vi "test2-ProcessAsyncMessageWithReplyInCSMLoop(SendAndReceive).vi"(8 "error in (no error)":errorcluster, 11 "TestCase in":refnum<class "testcase-CSMAddonLoopSupport.lvclass">) -> (0 "error out":errorcluster, 3 "TestCase out":refnum<class "testcase-CSMAddonLoopSupport.lvclass">)   [LabVIEW 2017, in "testcase-CSMAddonLoopSupport.lvclass"]
uses:
  testcase-CSMAddonLoopSupport.lvclass
  4585ddd5-ba69-4fd4-94fe-207595864cbd.vi
  a7620e19-6451-46a1-85ca-ade5edb58587.vi
  55fec5d7-cd22-46f7-b641-2c7c49619fc8.vi
  9cfd6824-310a-46c9-9b98-3854de5c7aa2.vi
  <vilib>/addons/_JKI Toolkits/VI Tester/TestCase.llb/TestCase.lvclass
  src/user.lib/_NEVSTOP/Communicable State Machine(CSM)/Communicable State Machine.lvlib
  CSM/CSM-Testcase.lvlib
  C:/Program Files (x86)/National Instruments/LabVIEW 2017/vi.lib/addons/_JKI Toolkits/VI Tester/TestCase.llb/TestCase.lvclass
panel:
  out "LoopCount":i32
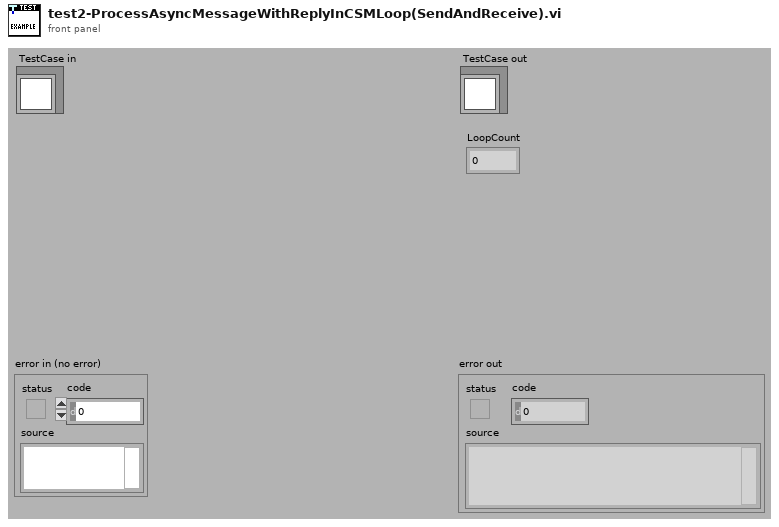
[diagram p1: front panel]
types:
  T1 = cluster{"Arguments":string, "Response":string, "error":errorcluster}
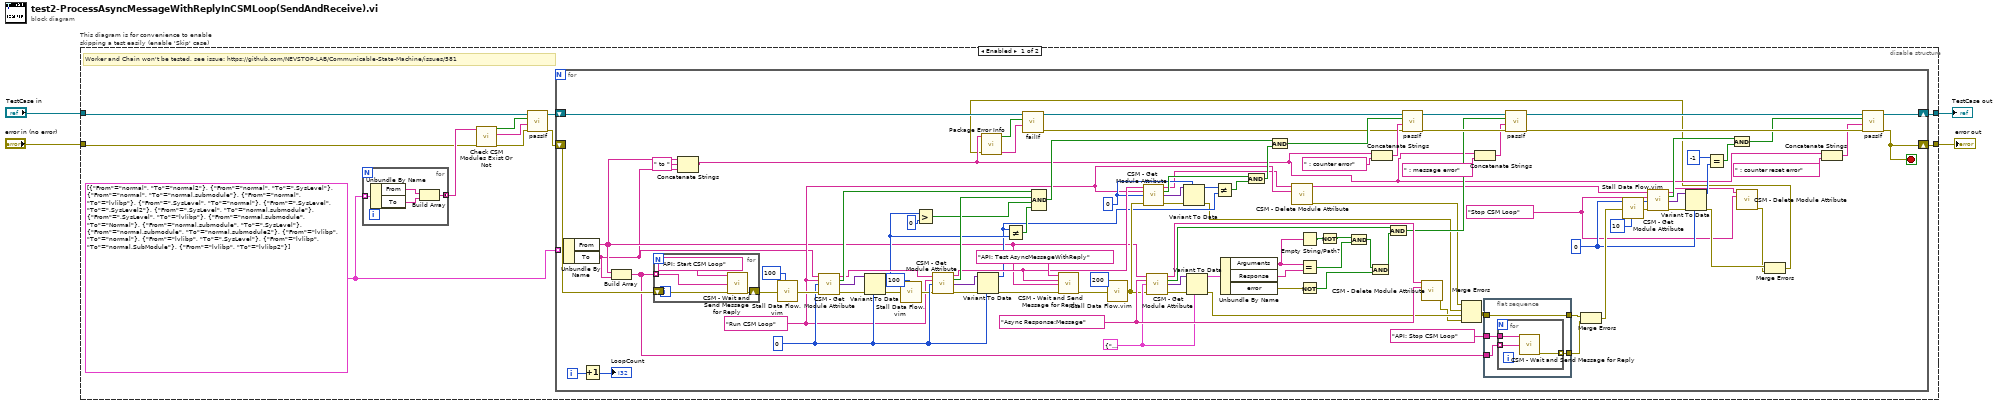
[diagram p0: block diagram]
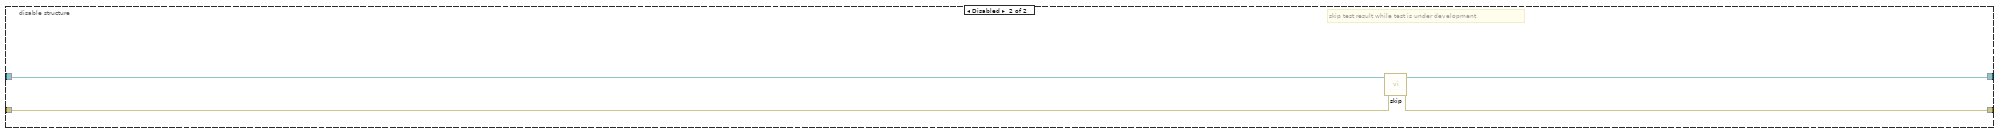
[diagram p2: hidden frame]
diagram:
  n1 = disable-structure "This diagram is for convenience to enable skipping a test easily (enable 'Skip' case)" shown="Enabled" {
    disable-tunnel: "TestCase in" -> [w6 w138]
    disable-tunnel: [w15 w136] -> w1
    disable-tunnel: [w14 w137] -> w3
    disable-tunnel: "error in (no error)" -> [w8 w135]
    frame Enabled {
      w9 = cluster{"From":string, "To":string}[] [{"From"="normal", "To"="normal2"}, {"From"="normal", "To"=".SysLevel"}, {"From"="normal", "To"="normal.submodule"}, {"From"="normal", "To"="lvlibp"}, {"From"=".SysLevel", "To"="normal"}, {"From"=".SysLevel", "To"=".SysLevel2"}, {"From"=".SysLevel", "To"="normal.submodule"}, {"From"=".SysLevel", "To"="lvlibp"}, {"From"="normal.submodule", "To"="Normal"}, {"From"="normal.submodule", "To"=".SysLevel"}, {"From"="normal.submodule", "To"="normal.submodule2"}, {"From"="lvlibp", "To"="normal"}, {"From"="lvlibp", "To"=".SysLevel"}, {"From"="lvlibp", "To"="normal.SubModule"}, {"From"="lvlibp", "To"="lvlibp2"}]
      # "Worker and Chain won't be tested, see issue: https://github.com/NEVSTOP-LAB/Communicable-State-Machine/issues/581"
      n2 = for {
        tunnel: w9 -> [w19] mode=indexing
        tunnel: [w16] -> w12 mode=concatenating
        n3 = Unbundle By Name(w19) -> ("From"=w18:string, "To"=w17:string)
        n4 = Build Array(w18, w17) -> (w16:string[])
      }
      n5 = call "Check CSM Modules Exist Or Not.vi"("error in"=w8, "CSM names in"=w12) -> ("error out"=w10:errorcluster, "Debug string"=w11:string, "All Modules Exist?"=w13:bool)  [unwired: 7 in]
      n6 = call-dynamic "passIf.vi"("error in (no error)"=w10, "message (\"\")"=w11, "pass"=w13, "TestCase in"=w6) -> ("error out"=w7:errorcluster, "TestCase out"=w5:refnum<class "testcase-CSMAddonLoopSupport.lvclass">)  [unwired: 6 in]
      n7 = for {
        tunnel: w9 -> [w39] mode=indexing
        shift-right: [w28] -> w15
        shift-left: w5 -> [w23]
        shift-right: [w27] -> w14
        shift-left: w7 -> [w65]
        i -> [w123]
        stop <- w27 stop-if-true
        w42 = "Stop CSM Loop" ("State")
        w55 = 0
        w75 = 0
        w90 = 0
        w46 = "Run CSM Loop" ("State")
        w101 = T1 {"Arguments"="", "Response"="", "error"={"status"=FALSE, "code"=0, "source"=""}}
        w102 = "Async Response:Message" ("State")
        n8 = Unbundle By Name(w39) -> ("From"=w37:string, "To"=w36:string)
        n9 = Increment(x=w123) -> (x+1=→"LoopCount":i32)
        n10 = Build Array(w37, w36) -> (w38:string[])
        n11 = for {
          shift-right: [w126] -> w121
          shift-left: w65 -> [w125]
          tunnel: w38 -> [w124] mode=indexing
          n12 = call "CSM - Wait and Send Message for Reply.vi"("State"="API: Start CSM Loop", "Target Module"=w124, "Error In (No Error)"=w125) -> ("error out"=w126:errorcluster)  [unwired: 9 in, 3 out]
        }
        n13 = Concatenate Strings(w37, " to " ("string"), w36) -> (w24:string)
        n14 = call "Stall Data Flow.vim"("value in"=w121, "milliseconds to wait"=u32 100) -> ("value out"=w98:errorcluster)  [unwired: 1 out]
        n15 = call "CSM - Get Module Attribute.vi"("CSM Name"=w36, "Attribute"=w46, "Default Value (Empty Variant)"=w90, "Error In"=w98) -> ("CSM Name (Dup)"=w92:string, "Found"=w97:bool, "Value"=w91:variant, "error out"=w95:errorcluster)  [unwired: 7 in, 1 out]
        n16 = Variant To Data(error in=w95, type=w90, Variant=w91) -> (data=w85:i32, error out=w84:errorcluster)
        n17 = call "Stall Data Flow.vim"("value in"=w84, "milliseconds to wait"=u32 100) -> ("value out"=w83:errorcluster)  [unwired: 1 out]
        n18 = Greater?(x=w85, y=0) -> (0:w88:bool)
        n19 = call "CSM - Get Module Attribute.vi"("CSM Name"=w92, "Attribute"=w46, "Default Value (Empty Variant)"=w90, "Error In"=w83) -> ("CSM Name (Dup)"=w80:string, "Found"=w96:bool, "Value"=w87:variant, "error out"=w94:errorcluster)  [unwired: 7 in, 1 out]
        n20 = Variant To Data(error in=w94, type=w90, Variant=w87) -> (data=w73:i32, error out=w93:errorcluster)
        n21 = Not Equal?(x=w73, y=w85) -> (x != y?=w86:bool)
        n22 = Compound Arithmetic op=AND(w97, w96, w88, w86) -> (w72:bool)
        n23 = call "CSM - Wait and Send Message for Reply.vi"("State"="API: Test AsyncMessageWithReply", "Arguments (\"\")"=w80, "Target Module"=w37, "Error In (No Error)"=w93) -> ("error out"=w117:errorcluster)  [unwired: 8 in, 3 out]
        n24 = call "Stall Data Flow.vim"("value in"=w117, "milliseconds to wait"=u32 200) -> ("value out"=w81:errorcluster)  [unwired: 1 out]
        n25 = call "CSM - Get Module Attribute.vi"("CSM Name"=w80, "Attribute"=w46, "Default Value (Empty Variant)"=w75, "Error In"=w81) -> ("CSM Name (Dup)"=w45:string, "Found"=w77:bool, "Value"=w76:variant, "error out"=w78:errorcluster)  [unwired: 7 in, 1 out]
        n26 = call "CSM - Get Module Attribute.vi"("CSM Name"=w37, "Attribute"=w102, "Default Value (Empty Variant)"=w101, "Error In"=w81) -> ("CSM Name (Dup)"=w110:string, "Found"=w112:bool, "Value"=w115:variant, "error out"=w116:errorcluster)  [unwired: 7 in, 1 out]
        n27 = Variant To Data(error in=w78, type=w75, Variant=w76) -> (data=w74:i32, error out=w44:errorcluster)
        n28 = Variant To Data(error in=w116, type=w101, Variant=w115) -> (data=w114:T1, error out=w100:errorcluster)
        n29 = Not Equal?(x=w74, y=w73) -> (x != y?=w79:bool)
        n30 = Unbundle By Name(w114) -> ("Arguments"=w105:string, "Response"=w104:string, "error"=w103:errorcluster)
        n31 = Compound Arithmetic op=AND(w77, w79) -> (w71:bool)
        n32 = And(x=w72, y=w71) -> (x .and. y?=w70:bool)
        n33 = call "CSM - Delete Module Attribute.vi"("CSM Name"=w45, "Attribute"=w46) -> ("CSM Name (Dup)"=w41:string, "error out"=w43:errorcluster)  [unwired: 10 in, 2 out]
        n34 = Empty String/Path?(string/path=w105) -> (empty?=w109:bool)
        n35 = Equal?(x=w105, y=w104) -> (x = y?=w107:bool)
        n36 = Not(x=w103) -> (.not. x?=w113:bool)
        n37 = Not(x=w109) -> (.not. x?=w108:bool)
        n38 = And(x=w108, y=w107) -> (x .and. y?=w106:bool)
        n39 = And(x=w106, y=w113) -> (x .and. y?=w111:bool)
        n40 = Concatenate Strings(w24, " : counter error" ("format string")) -> (w33:string)
        n41 = And(x=w112, y=w111) -> (x .and. y?=w67:bool)
        n42 = call "CSM - Delete Module Attribute.vi"("CSM Name"=w110, "Attribute"=w102) -> ("error out"=w99:errorcluster)  [unwired: 10 in, 3 out]
        n43 = Merge Errors(w43, w44, w100, w99) -> (w47:errorcluster)
        n44 = Concatenate Strings(w24, " : message error" ("format string")) -> (w31:string)
        n45 = flat-sequence {
          tunnel: "API: Stop CSM Loop" ("State") -> [w131]
          tunnel: [w130] -> w62
          tunnel: [w129] -> w48
          tunnel: w47 -> [w129]
          tunnel: w38 -> [w128]
          frame #0 {
            n46 = for {
              tunnel: w131 -> [w134]
              tunnel: [w133] -> w130 mode=indexing
              tunnel: w128 -> [w132] mode=indexing
              n47 = call "CSM - Wait and Send Message for Reply.vi"("State"=w134, "Target Module"=w132) -> ("error out"=w133:errorcluster)  [unwired: 10 in, 3 out]
            }
          }
        }
        n48 = Merge Errors(w48, w62) -> (w60:errorcluster)
        n49 = call "Stall Data Flow.vim"("value in"=w60, "milliseconds to wait"=u32 10) -> ("value out"=w59:errorcluster)  [unwired: 1 out]
        n50 = call "CSM - Get Module Attribute.vi"("CSM Name"=w41, "Attribute"=w42, "Default Value (Empty Variant)"=w55, "Error In"=w59) -> ("CSM Name (Dup)"=w40:string, "Found"=w58:bool, "Value"=w56:variant, "error out"=w57:errorcluster)  [unwired: 7 in, 1 out]
        n51 = Variant To Data(error in=w57, type=w55, Variant=w56) -> (data=w54:i32, error out=w50:errorcluster)
        n52 = Equal?(x=-1, y=w54) -> (x = y?=w51:bool)
        n53 = And(x=w58, y=w51) -> (x .and. y?=w52:bool)
        n54 = call "CSM - Delete Module Attribute.vi"("CSM Name"=w40, "Attribute"=w42) -> ("error out"=w49:errorcluster)  [unwired: 10 in, 3 out]
        n55 = Merge Errors(w50, w49) -> (w20:errorcluster)
        n56 = call "Package Error Info.vi"("error in"=w20, "String in"=w24) -> ("packed error info out"=w25:string, "error status"=w26:bool)  [unwired: 8 in]
        n57 = call-dynamic "failIf.vi"("message (\"\")"=w25, "fail"=w26, "TestCase in"=w23) -> ("error out"=w21:errorcluster, "TestCase out"=w22:refnum<class "testcase-CSMAddonLoopSupport.lvclass">)  [unwired: 7 in]
        n58 = call-dynamic "passIf.vi"("error in (no error)"=w21, "message (\"\")"=w33, "pass"=w70, "TestCase in"=w22) -> ("error out"=w68:errorcluster, "TestCase out"=w69:refnum<class "testcase-CSMAddonLoopSupport.lvclass">)  [unwired: 6 in]
        n59 = call-dynamic "passIf.vi"("error in (no error)"=w68, "message (\"\")"=w31, "pass"=w67, "TestCase in"=w69) -> ("error out"=w63:errorcluster, "TestCase out"=w64:refnum<class "testcase-CSMAddonLoopSupport.lvclass">)  [unwired: 6 in]
        n60 = Concatenate Strings(w24, " : counter reset error" ("format string")) -> (w29:string)
        n61 = call-dynamic "passIf.vi"("error in (no error)"=w63, "message (\"\")"=w29, "pass"=w52, "TestCase in"=w64) -> ("error out"=w27:errorcluster, "TestCase out"=w28:refnum<class "testcase-CSMAddonLoopSupport.lvclass">)  [unwired: 6 in]
      }
    }
    frame Disabled {
      # "skip test result while test is under development"
      n62 = call <vilib>:"skip.vi"("error in (no error)"=w135, "TestCase in"=w138) -> ("error out"=w137:errorcluster, "TestCase out"=w136:refnum<class "testcase-CSMAddonLoopSupport.lvclass">)  [unwired: 8 in]
    }
  }
  "error out" <- w3
  "TestCase out" <- w1
